vi "KM101_SetChannelEnable.vi"(9 "使能模式":T1(ring), 10 "reference in":refnum<k7>) -> (2 "reference out":refnum<k7>)   [LabVIEW 2018, in "KIM101lib.lvlib"]
uses:
  KIM101lib.lvlib
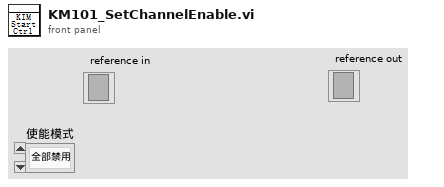
[diagram p1: front panel]
types:
  T1 = enum16{"全部禁用", "CH1使能", "CH2使能", "CH3使能", "CH4使能", "CH1,CH2使能", "CH3,CH4使能"}
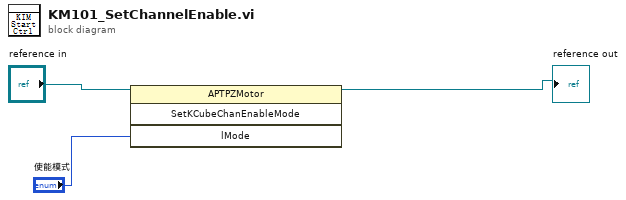
[diagram p0: block diagram]
diagram:
  n1 = invoke class="APTPZMotor" method="SetKCubeChanEnableMode"(reference="reference in", "lMode"="使能模式") -> (reference out=→"reference out":refnum<k7>)  [unwired: 2 in, 3 out]
